vi "MajorMinorAxes.vi"(9 "Best Fits":dbl[](array[numeric]), 10 "Image in":T2) -> (2 "cross lines":T1)   [LabVIEW 2015]
uses:
  <vilib>/vision/Image Controls.llb/IMAQ Image.ctl
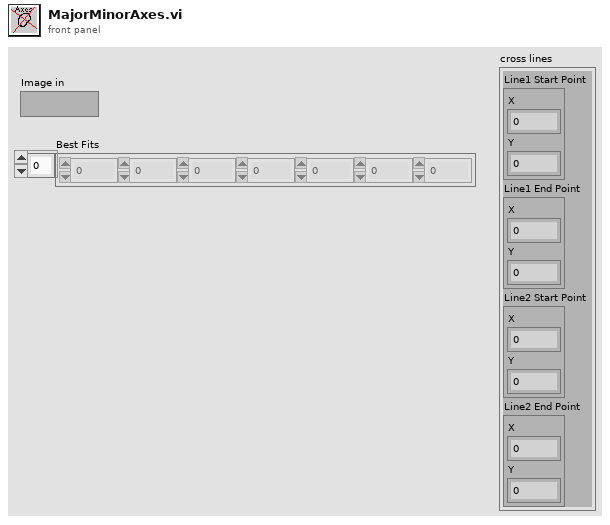
[diagram p1: front panel]
types:
  T1 = cluster{"Line1 Start Point":cluster{"X":i32, "Y":i32}, "Line1 End Point":cluster{"X":i32, "Y":i32}, "Line2 Start Point":cluster{"X":i32, "Y":i32}, "Line2 End Point":cluster{"X":i32, "Y":i32}}
  T2 = typedef "IMAQ Image.ctl" = refnum<image>
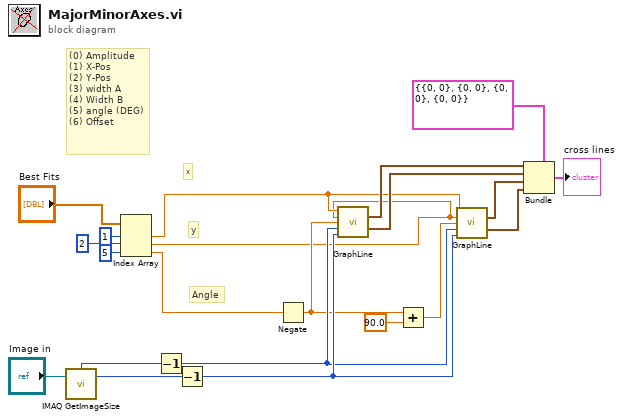
[diagram p0: block diagram]
diagram:
  # "Angle"
  # "y"
  # "x"
  # "(0) Amplitude\n(1) X-Pos\n(2) Y-Pos\n(3) width A\n(4) Width B\n(5) angle (DEG)\n(6) Offset"
  n1 = call "IMAQ GetImageSize"("Image"="Image in") -> ("Y Resolution"=w15:i32, "X Resolution"=w16:i32)  [unwired: 3 in, 1 out]
  n2 = Index Array(array="Best Fits", index #1=1 ("index"), index #2=2 ("index"), index #3=5 ("index")) -> (element #1=w3:dbl, element #2=w2:dbl, element #3=w1:dbl)
  n3 = Decrement(x=w16) -> (x-1=w20:i32)
  n4 = Decrement(x=w15) -> (x-1=w21:i32)
  n5 = Negate(x=w1) -> (-x=w18:dbl)
  n6 = call "GraphLine.vi"("xp"=w3, "yp"=w2, "alpha"=w18, "xmax"=w20, "ymax"=w21) -> ("Start Point"=w13:cluster{"X":i32, "Y":i32}, "End Point"=w12:cluster{"X":i32, "Y":i32})  [unwired: 9 in]
  n7 = Add(x=w18, y=90.0) -> (x+y=w19:dbl)
  n8 = call "GraphLine.vi"("xp"=w3, "yp"=w2, "alpha"=w19, "xmax"=w20, "ymax"=w21) -> ("Start Point"=w11:cluster{"X":i32, "Y":i32}, "End Point"=w10:cluster{"X":i32, "Y":i32})  [unwired: 9 in]
  n9 = Bundle(cluster=T1 {"Line1 Start Point"={"X"=0, "Y"=0}, "Line1 End Point"={"X"=0, "Y"=0}, "Line2 Start Point"={"X"=0, "Y"=0}, "Line2 End Point"={"X"=0, "Y"=0}}, "Line1 Start Point"=w13, "Line1 End Point"=w12, "Line2 Start Point"=w11, "Line2 End Point"=w10) -> (→"cross lines":T1)
